vi "SLSC Unpack FIFO Command.vi"(11 "SPI CMD FIFO Element":u64) -> (0 "Data to DAC":u64, 1 "Chip Select":u8, 2 "CS Bit Value/Slot #":u8, 3 "Transfer Length":u8, 5 "Rack #":u8)   [LabVIEW 2014, in "SLSC FPGA Toolkit.lvlib"]
uses:
  SLSC FPGA Toolkit.lvlib
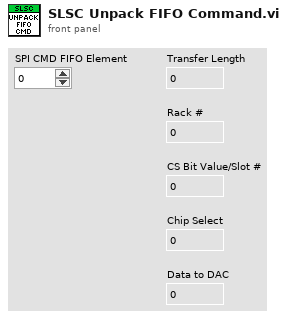
[diagram p1: front panel]
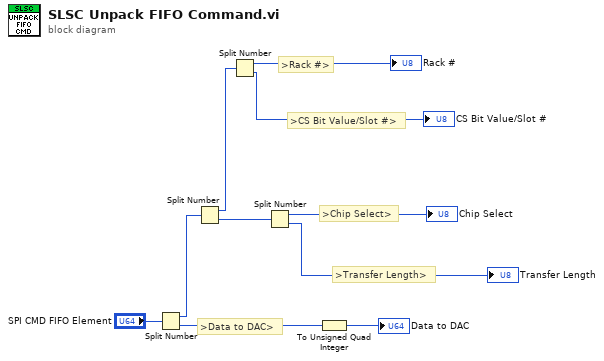
[diagram p0: block diagram]
diagram:
  # ">CS Bit Value/Slot #>"
  # ">Transfer Length>"
  # ">Rack #>"
  # ">Data to DAC>"
  # ">Chip Select>"
  n1 = Split Number(x="SPI CMD FIFO Element") -> (hi(x)=w2:u32, lo(x)=w1:u32)
  n2 = Split Number(x=w2) -> (hi(x)=w5:u16, lo(x)=w3:u16)
  n3 = Split Number(x=w5) -> (hi(x)=→"Rack #":u8, lo(x)=→"CS Bit Value/Slot #":u8)
  n4 = Split Number(x=w3) -> (hi(x)=→"Chip Select":u8, lo(x)=→"Transfer Length":u8)
  n5 = To Unsigned Quad Integer(1:w1) -> (0:→"Data to DAC":u64)
